vi "1L04-tb1D-Rech-F(y)_de_y.vi"(1 "y":dbl, 2 "F(x)":dbl[](array[numeric]), 3 "x":dbl[](array[numeric])) -> (0 "F(y) interpolé":dbl)   [LabVIEW 2010, in "lv_01.lvlib"]
doc: "Soit en entrée les tableaux 1D x et F(x), le VI retourne la valeur F(y) pour y en entrée. \nTraitement par interpolation même si la valeur de y n'a pas de correspondance dans le tableau x"
uses:
  lv_01.lvlib
panel:
  # "Identifier / Utiliser"
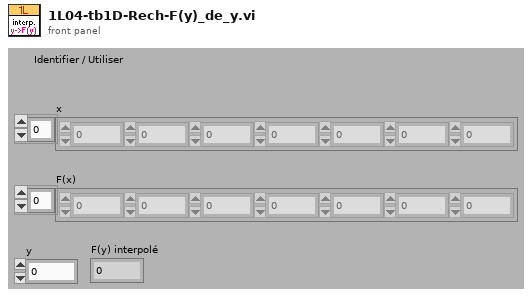
[diagram p1: front panel]
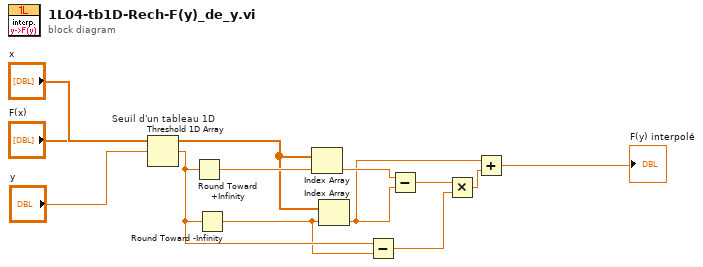
[diagram p0: block diagram]
diagram:
  n1 = Threshold 1D Array "Seuil d'un tableau 1D"(2:"y", 3:"x") -> (0:w5:dbl)  [unwired: 1 in]
  n2 = Round Toward +Infinity(x=w5) -> (ceil(x): smallest int >= x=w11:dbl)
  n3 = Round Toward -Infinity(1:w5) -> (0:w4:dbl)
  n4 = Index Array(array="F(x)", index=w11) -> (element=w10:dbl)
  n5 = Index Array(array="F(x)", index=w4) -> (element=w7:dbl)
  n6 = Subtract(x=w5, y=w4) -> (x-y=w3:dbl)
  n7 = Subtract(x=w10, y=w7) -> (x-y=w9:dbl)
  n8 = Multiply(x=w9, y=w3) -> (x*y=w8:dbl)
  n9 = Add(x=w7, y=w8) -> (x+y=→"F(y) interpolé":dbl)
